vi "quit trial.vi"   [LabVIEW 2018]
uses:
  <vilib>/rvi/interface/nirviOpenFPGA/nirviOpenFPGA.xnode
  FPGA Bitfiles/CompressorRigV2_CompressorFPGA_FPGAMain_VETZPGqYdEE.lvbitx
  Queue VIs/En-queue RT data element.vi
  <vilib>/FPGAPlugInAG/cRIO-9056/niLvFpga_Open_cRIO-9056.vi
  <vilib>/rvi/interface/common/dynamic/niFpgaDynamicAddResources.vi
types:
  T1 = typedef "Message loop data.ctl" = cluster{"Parameters":cluster{"FPGA Ref":T2, "configID":u32, "activeChannels":cluster{"index":u16, "name":string}[]}, "Variables":cluster{"RT Status":T3, "watchdog":timestamp, "limitsEnabled":bool, "Interlocks":cluster{"gearboxOil":bool, "bearingOil":bool, "gearboxAir":bool}}}
  T2 = typedef "FPGA reference.ctl" = refnum<k20>
  T3 = typedef "RT Status.ctl" = cluster{"Comms loop":bool, "scheduler loop":bool, "data process loop":bool, "FIFO loop":bool, "Command Stream":bool, "Error Stream":bool, "FPGA FIFO":bool, "Data Stream":bool}
  T4 = typedef "Analogue loop data.ctl" = cluster{"Params":cluster{"FPGA ref":T2, "Total Channels":u32}, "Variables":cluster{"FIFO wait counter":u16, "FIFO read trigger":u32}}
  T5 = typedef "comms data.ctl" = cluster{"Parameters":cluster{"error writer name":string, "command reader name":string, "error buffer size":i32, "command buffer size":i32, "scanivalveIP":string, "scanivalvePeriod":u16}, "Variables":cluster{"listen schedule":u32, "incident buffer":T6[], "command stream":refnum<k21>, "error stream":refnum<k21>, "waiting for command stream connect":bool, "waiting for error stream connect":bool, "scanivalve connection":refnum<k5>, "scanivalveScheduleID":u32, "activeScanivalvePorts":i32[], "channelCount":i16}, "scanivalveConfig":T7}
  T6 = typedef "generic incident.ctl" = cluster{"timestamp":timestamp, "type":string, "Variant":variant}
  T7 = typedef "Scanivalve API.lvlib/scanivalveConfig.ctl" = cluster{"listS":T8, "listC":T9, "listSG":T10, "activeChannels":T11}
  T8 = typedef "Scanivalve API.lvlib/listS.ctl" = cluster{"period":u16, "ADtrig":bool, "ScanTrig":bool, "page":u16, "qpkts":u16}
  T9 = typedef "Scanivalve API.lvlib/listC.ctl" = cluster{"ZC":bool, "unitScan":string, "CvtUnit":dbl, "bin":bool, "EU":bool}
  T10 = typedef "Scanivalve API.lvlib/listSG.ctl" = cluster{"Avg1":u16, "FPS1":u16, "SGEnable1":bool}
  T11 = typedef "Scanivalve API.lvlib/chan1.ctl" = cluster{"Chan1":cluster{"101":bool, "102":bool, "103":bool, "104":bool, "109":bool, "110":bool, "111":bool, "112":bool, "201":bool, "202":bool, "203":bool, "204":bool, "209":bool, "210":bool, "211":bool, "212":bool, "301":bool, "302":bool, "303":bool, "304":bool, "309":bool, "310":bool, "311":bool, "312":bool, "401":bool, "402":bool, "403":bool, "404":bool, "409":bool, "410":bool, "411":bool, "412":bool}}
  T12 = typedef "Data processing loop data.ctl" = cluster{"Parameters":cluster{"FPGA Ref":T2, "data stream":cluster{"data writer name":string, "NS write buffer size":i32, "NS Buffer length":u32}, "FIFO Depth":u32, "Channel controls":cluster{"FIFO channel count":i32, "active indices":i16[], "active channels":i32, "channelScaling":T13[], "scanivalveCount":i32, "channels":refnum<class "Data Channel.lvclass">[]}, "safetyChannels":cluster{"oilP":u16, "airP":u16, "water":u16, "channelLimits":T16[]}, "speedChannel":i32, "maxSpeedLimit":dbl, "Torque":cluster{"fixedOffset":dbl, "filter":bool, "fallingEdge":bool, "swapEncoders":bool}}, "Variables":cluster{"Intermediary buffer":dbl[][], "buffer position":u32, "write loop counter":u16, "NS write trigger":u32, "NS Connection status":bool, "waiting for NS":bool, "labAmbient":cluster{"pressure":dbl, "temperature":dbl}, "scanivalvePorts":u16[], "scanivalvePressures":dbl[], "data stream":refnum<k21>, "activeChannelLimitIndex":u16[], "runningSpeedLimit":dbl, "speedChannelIndex":i32, "Interlocks":cluster{"gearboxOil":bool, "bearingOil":bool, "gearboxAir":bool}, "interlockChannels":cluster{"gearboxOil":i32, "bearingOil":i32, "air":i32}, "limitStates":cluster{"warn":bool, "alarm":bool}[]}}
  T13 = typedef "channelControl.ctl" = cluster{"index":u16, "active":bool, "channelType":T14, "module":u16, "terminal":u16, "channelName":string, "scalingMethod":T15, "scalingParameters":dbl[], "scaledUnits":string, "tempOffset":dbl}
  T14 = typedef "channelScalingTypes.ctl" = enum16{"calculation", "measurement", "scanivalve", "output", "digital"}
  T15 = typedef "scalingMethods.ctl" = enum16{"none", "linear", "thermocouple", "polynomial", "encoder", "RTD"}
  T16 = typedef "channelLimitControl.ctl" = cluster{"channelID":u16, "Enabled":bool, "warnValue":dbl, "limitValue":dbl, "Invert":bool, "limitAction":T17}
  T17 = typedef "limitActions.ctl" = enum16{"stop", "shutdown", "ignore"}
  T18 = cluster{"Message":T1, "FIFO":T4, "Comms data":T5, "Data processor":T12}
  T19 = typedef "Queues cluster.ctl" = cluster{"RT Message":refnum<queue>, "RT Comms":refnum<queue>, "RT Data":refnum<queue>, "RT FIFO":refnum<queue>, "message scheduler":refnum<class "message scheduler.lvclass">}
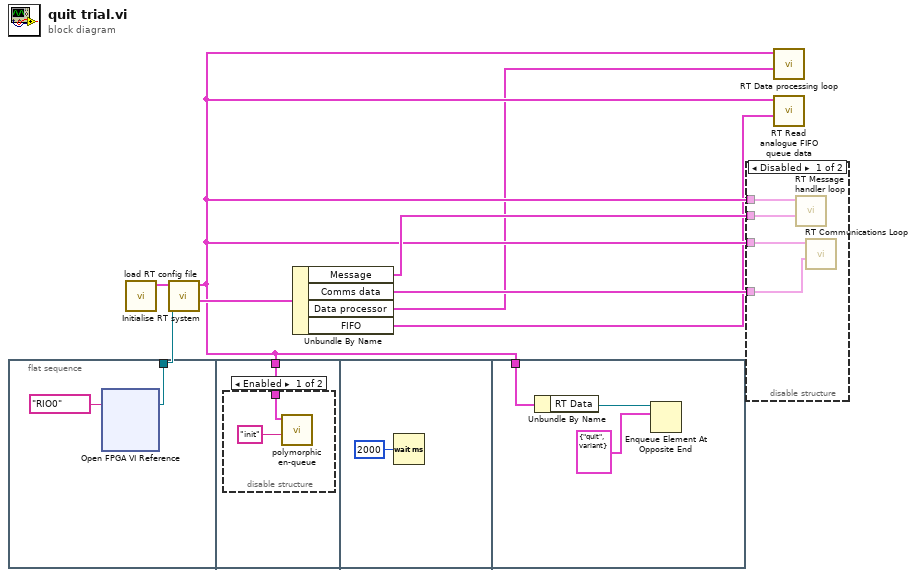
[diagram p0: block diagram]
diagram:
  n1 = flat-sequence {
    tunnel: [w9] -> w7
    tunnel: w3 -> [w11]
    tunnel: w3 -> [w17]
    frame #0 {
      n2 = xnode "Open FPGA VI Reference"("resource name"=tag "RIO0") -> ("FPGA VI Reference Out"=w9:refnum<k20>)  [unwired: 1 in, 1 out]
    }
    frame #1 {
      n3 = disable-structure shown="Enabled" {
        disable-tunnel: w11 -> [w13 _]
        frame Enabled {
          n4 = call-poly "polymorphic en-queue.vi"("Message"="init", "RT Queues"=w13) -> ()  [unwired: 7 in, 3 out]
        }
        frame Disabled {
        }
      }
    }
    frame #2 {
      n5 = Wait (ms)(milliseconds to wait=u32 2000) -> ()  [unwired: 1 out]
    }
    frame #3 {
      n6 = Unbundle By Name(w17) -> ("RT Data"=w16:refnum<queue>)
      n7 = Enqueue Element At Opposite End(queue=w16, element=cluster{"Message":string, "Data":variant} {"Message"="quit", "Data"=variant}) -> ()  [unwired: 2 in, 3 out]
    }
  }
  n8 = call "load RT config file.vi"() -> ("config data out"=w6:T18)  [unwired: 8 in, 3 out]
  n9 = call "Initialise RT system.vi"("CompressorRigV2"=w7, "config data out"=w6) -> ("config data"=w8:T18, "Queues"=w3:T19)  [unwired: 8 in]
  n10 = Unbundle By Name(w8) -> ("Message"=w5:T1, "Comms data"=w4:T5, "Data processor"=w1:T12, "FIFO"=w2:T4)
  n11 = disable-structure shown="Disabled" {
    disable-tunnel: w5 -> [w21 _]
    disable-tunnel: w3 -> [w20 _]
    disable-tunnel: w4 -> [w19 _]
    disable-tunnel: w3 -> [w18 _]
    frame Disabled {
      n12 = call "RT Message handler loop.vi"("Message handler data"=w21, "RT Queues"=w20) -> ()  [unwired: 9 in, 1 out]
      n13 = call "RT Communications Loop.vi"("Comms data"=w19, "RT Queues"=w18) -> ()  [unwired: 10 in]
    }
    frame Enabled {
    }
  }
  n14 = call "RT Data processing loop.vi"("Data"=w1, "RT Queues"=w3) -> ()  [unwired: 10 in]
  n15 = call "RT Read analogue FIFO queue data.vi"("FIFO parameters"=w2, "RT Queues"=w3) -> ()  [unwired: 10 in]
